vi "matrix-multiply-benchmark.vi"() -> ()   [LabVIEW 2019]
uses:
  <vilib>/Analysis/Matrix/Datatypes/RealMatrix.ctl
  <vilib>/Analysis/baseanly.llb/Real A x B.vi
  <vilib>/Analysis/Matrix/Numeric/Add/Add (Elementwise) - RM,R.vi
  <vilib>/Analysis/Matrix/Numeric/Multiply/Multiply - RM,R.vi
  <vilib>/Analysis/Matrix/Numeric/Multiply/Multiply - RM,RM.vi
  <vilib>/Rock Robotics/WPI/ThirdParty/JAS_Junk/TrajLib/Trajectory_Library.lvlib
  <vilib>/Analysis/Matrix/NI_Matrix.lvlib
  <vilib>/Analysis/NI_AALBase.lvlib
  <vilib>/Analysis/Matrix/Comparison/Equal/Equal - RM,RM.vi
panel:
  out "A = B?":bool
  out "B c":i32
  out "B r":i32
  out "A c":i32
  out "A r":i32
  out "lin alg add removed":dbl
  out "mtraix add removed":dbl
  out "output matrix":T1
  out "linalg":T1
  out "mat xpose":T1
  out "Add only":dbl format="%18.3f"
  out "LinearAlg Mult":dbl format="%18.3f"
  out "Matrix Mult":dbl format="%18.3f"
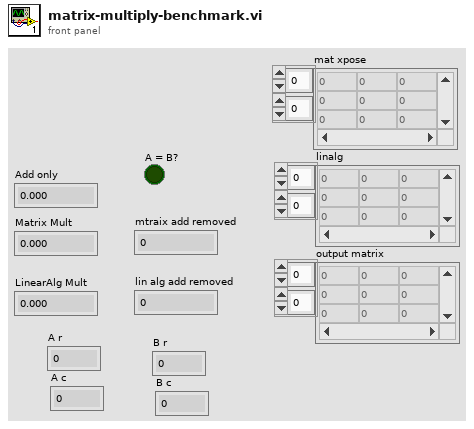
[diagram p1: front panel]
types:
  T1 = typedef "NI_Matrix.lvlib/RealMatrix.ctl" = dbl[][]
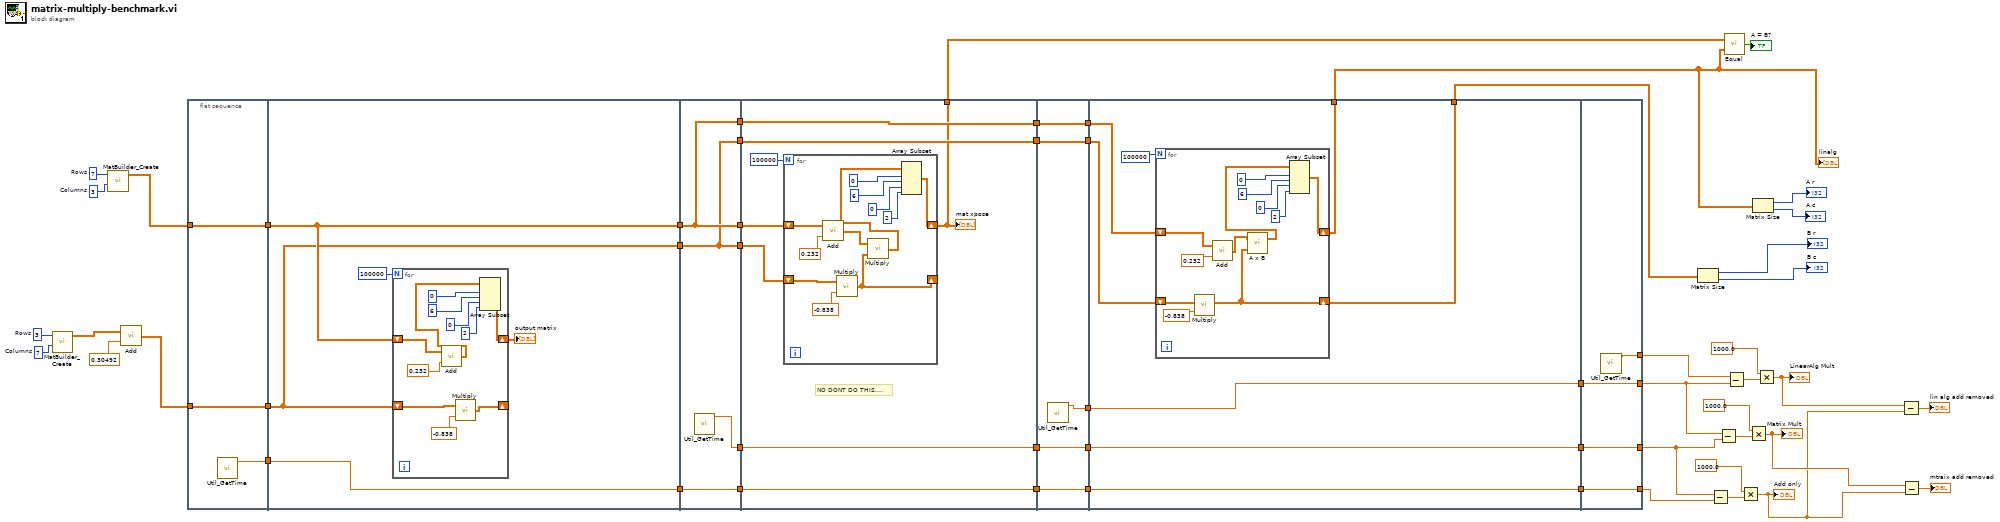
[diagram p0: block diagram]
diagram:
  w18 = 7  # Columns
  w19 = 3  # Rows
  w44 = 3  # Columns
  w45 = 7  # Rows
  n1 = call <vilib>:"MatBuilder_Create.vi"("Columns"=w18, "Rows"=w19) -> ("output matrix"=w10:T1)  [unwired: 9 in]
  n2 = call <vilib>:"MatBuilder_Create.vi"("Columns"=w44, "Rows"=w45) -> ("output matrix"=w43:T1)  [unwired: 9 in]
  n3 = call-poly <vilib>:"Add.vi"("Real Scalar c"=0.30492, "Real Matrix A"=w10) -> ("A + c"=w11:T1)
  n4 = flat-sequence {
    tunnel: w43 -> [w58]
    tunnel: [w58] -> w37
    tunnel: [w57] -> w29
    tunnel: [w56] -> w17
    tunnel: w11 -> [w56]
    tunnel: [w61] -> w38
    tunnel: w37 -> [w61]
    tunnel: [w63] -> w30
    tunnel: w29 -> [w63]
    tunnel: w17 -> [w59]
    tunnel: [w59] -> w15
    tunnel: [w78] -> w55
    tunnel: [w77] -> w42
    tunnel: [w77] -> w39
    tunnel: w38 -> [w77]
    tunnel: [w76] -> w31
    tunnel: w30 -> [w76]
    tunnel: [w75] -> w16
    tunnel: w15 -> [w75]
    tunnel: [w75] -> w13
    tunnel: w55 -> [w86]
    tunnel: [w86] -> w54
    tunnel: w42 -> [w84]
    tunnel: [w83] -> w40
    tunnel: w39 -> [w83]
    tunnel: [w82] -> w32
    tunnel: w31 -> [w82]
    tunnel: w16 -> [w81]
    tunnel: [w80] -> w14
    tunnel: w13 -> [w80]
    tunnel: [w79] -> w1
    tunnel: w54 -> [w102]
    tunnel: [w103] -> w51
    tunnel: [w102] -> w46
    tunnel: [w101] -> w41
    tunnel: w40 -> [w101]
    tunnel: [w100] -> w33
    tunnel: w32 -> [w100]
    tunnel: w14 -> [w99]
    tunnel: [w99] -> w12
    tunnel: w51 -> [w111]
    tunnel: [w111] -> w48
    tunnel: [w110] -> w47
    tunnel: w46 -> [w110]
    tunnel: w41 -> [w108]
    tunnel: [w107] -> w34
    tunnel: w33 -> [w107]
    tunnel: w12 -> [w106]
    tunnel: [w105] -> w3
    tunnel: [w104] -> w4
    tunnel: [w127] -> w36
    tunnel: [w126] -> w35
    tunnel: w48 -> [w126]
    tunnel: [w125] -> w26
    tunnel: w47 -> [w125]
    tunnel: [w124] -> w25
    tunnel: w34 -> [w124]
    frame #0 {
      n5 = call <vilib>:"Util_GetTime.vi"() -> ("FPGA_Time_Seconds"=w57:dbl)  [unwired: 10 in, 1 out]
    }
    frame #1 {
      n6 = for {
        N: 100000 -> [_]
        shift-right: [w64] -> w60
        shift-left: w61 -> [w73]
        shift-right: [w70] -> _
        shift-left: w59 -> [w71]
        n7 = call-poly <vilib>:"Add.vi"("Real Scalar c"=0.232, "Real Matrix A"=w73) -> ("A + c"=w65:T1)
        n8 = call-poly <vilib>:"Multiply.vi"("Real Scalar c"=-0.838, "Real Matrix A"=w71) -> ("A * c"=w70:T1)
        n9 = Array Subset(array=w65, index (row)=0 ("row 1"), length (row)=6 ("row N"), index (col)=0 ("column 1"), length (col)=2 ("column N")) -> (w64:T1)
      }
      "output matrix" <- w60
    }
    frame #2 {
      n10 = call <vilib>:"Util_GetTime.vi"() -> ("FPGA_Time_Seconds"=w78:dbl)  [unwired: 10 in, 1 out]
    }
    frame #3 {
      # "NO DONT DO THIS...."
      n11 = for {
        N: 100000 -> [_]
        shift-right: [w88] -> w79
        shift-left: w84 -> [w93]
        shift-right: [w95] -> _
        shift-left: w81 -> [w96]
        n12 = call-poly <vilib>:"Add.vi"("Real Scalar c"=0.232, "Real Matrix A"=w93) -> ("A + c"=w94:T1)
        n13 = call-poly <vilib>:"Multiply.vi"("Real Scalar c"=-0.838, "Real Matrix A"=w96) -> ("A * c"=w95:T1)
        n14 = call-poly <vilib>:"Multiply.vi"("Real Matrix B"=w95, "Real Matrix A"=w94) -> ("A * B"=w87:T1)
        n15 = Array Subset(array=w87, index (row)=0 ("row 1"), length (row)=6 ("row N"), index (col)=0 ("column 1"), length (col)=2 ("column N")) -> (w88:T1)
      }
      "mat xpose" <- w79
    }
    frame #4 {
      n16 = call <vilib>:"Util_GetTime.vi"() -> ("FPGA_Time_Seconds"=w103:dbl)  [unwired: 10 in, 1 out]
    }
    frame #5 {
      n17 = for {
        N: 100000 -> [_]
        shift-right: [w112] -> w105
        shift-left: w108 -> [w120]
        shift-right: [w118] -> w104
        shift-left: w106 -> [w121]
        n18 = call-poly <vilib>:"Multiply.vi"("Real Scalar c"=-0.838, "Real Matrix A"=w121) -> ("A * c"=w118:T1)
        n19 = call-poly <vilib>:"Add.vi"("Real Scalar c"=0.232, "Real Matrix A"=w120) -> ("A + c"=w119:T1)
        n20 = call-poly <vilib>:"A x B.vi"("B"=w118, "A"=w119) -> ("A x B"=w113:T1)  [unwired: 1 out]
        n21 = Array Subset(array=w113, index (row)=0 ("row 1"), length (row)=6 ("row N"), index (col)=0 ("column 1"), length (col)=2 ("column N")) -> (w112:T1)
      }
    }
    frame #6 {
      n22 = call <vilib>:"Util_GetTime.vi"() -> ("FPGA_Time_Seconds"=w127:dbl)  [unwired: 10 in, 1 out]
    }
  }
  n23 = Matrix Size(0:w4) -> (1:→"B r":i32, 2:→"B c":i32)
  n24 = Subtract(x=w26, y=w25) -> (x-y=w28:dbl)
  n25 = Subtract(x=w35, y=w26) -> (x-y=w53:dbl)
  n26 = call-poly <vilib>:"Equal.vi"("Real Matrix B"=w3, "Real Matrix A"=w1) -> ("A = B?"=→"A = B?":bool)
  n27 = Subtract(x=w36, y=w35) -> (x-y=w50:dbl)
  n28 = Multiply(x=1000.0, y=w28) -> (x*y=w22:dbl)
  "Add only" <- w22
  n29 = Multiply(x=1000.0, y=w53) -> (x*y=w23:dbl)
  "Matrix Mult" <- w23
  n30 = Matrix Size(0:w3) -> (1:→"A r":i32, 2:→"A c":i32)
  n31 = Multiply(x=1000.0, y=w50) -> (x*y=w24:dbl)
  "LinearAlg Mult" <- w24
  n32 = Subtract(x=w24, y=w22) -> (x-y=→"lin alg add removed":dbl)
  n33 = Subtract(x=w23, y=w22) -> (x-y=→"mtraix add removed":dbl)
  "linalg" <- w3
